vi "Read SelfQueue.vi"(8 "error in (no error)":errorcluster, 11 "ModuleAbstract in":refnum<class "ModuleAbstract.lvclass">) -> (0 "error out":errorcluster, 2 "SelfQueue":refnum<queue>, 3 "ModuleAbstract out":refnum<class "ModuleAbstract.lvclass">)   [LabVIEW 2019, in "ModuleAbstract.lvlib" / "ModuleAbstract.lvclass"]
uses:
  ModuleAbstract.lvclass
  Utilities/LV_Lib/Message Queue/Message Cluster.ctl
  Utilities/LV_Lib/Message Queue/Message Queue.lvlib
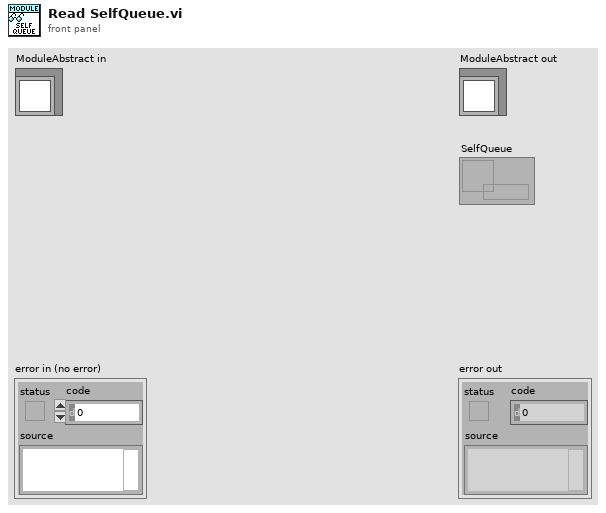
[diagram p1: front panel]
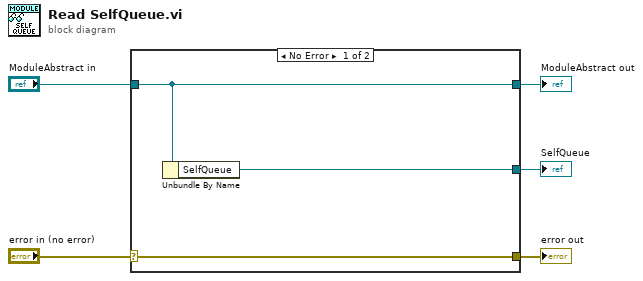
[diagram p0: block diagram]
diagram:
  n1 = case shown="No Error" "error in (no error)" {
    selector: "error in (no error)" -> [w8 w9]
    tunnel: [w8 w9] -> w4
    tunnel: [w7 w10] -> w2
    tunnel: "ModuleAbstract in" -> [w7 w10]
    tunnel: [w6 _] -> w1
    frame No Error {
      n2 = Unbundle By Name(w7) -> ("SelfQueue"=w6:refnum<queue>)
    }
    frame Error {
    }
  }
  "error out" <- w4
  "ModuleAbstract out" <- w2
  "SelfQueue" <- w1
